vi "Enc_real.vi"(1 "Command":i32, 2 "Encoder":i32, 3 "Encoder_real_in":i32) -> (0 "Encoder_real_out":i32)   [LabVIEW 2015]
panel:
  out "XOR":bool
  out "Cmd > 0?":bool
  out "E(t)-E(t-1)":i32
  out "E(t)-E(t-1) > 0?":bool
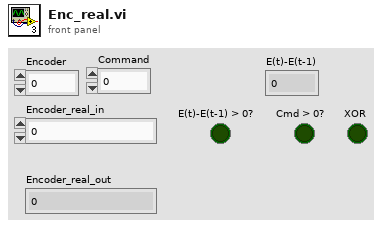
[diagram p1: front panel]
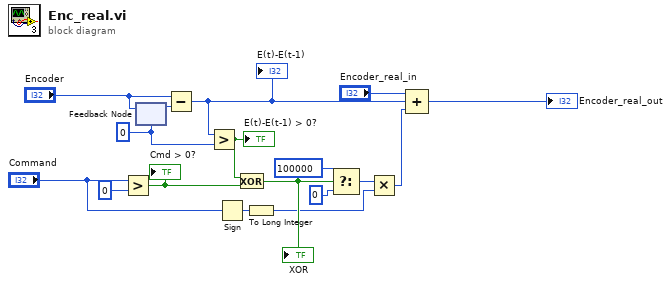
[diagram p0: block diagram]
diagram:
  w17 = 0
  n1 = Greater?(x="Command", y=0) -> (0:w15:bool)
  "Cmd > 0?" <- w15
  n2 = feedback #1(w17) -> (w2:i32)
  n3 = feedback-in #1("Encoder") -> ()
  n4 = Subtract(x="Encoder", y=w2) -> (x-y=w6:i32)
  "E(t)-E(t-1)" <- w6
  n5 = Greater?(x=w6, y=w17) -> (0:w16:bool)
  "E(t)-E(t-1) > 0?" <- w16
  n6 = Sign(1:"Command") -> (0:w12:i32)
  n7 = Exclusive Or(1:w15, 2:w16) -> (0:w14:bool)
  "XOR" <- w14
  n8 = To Long Integer(number=w12) -> (32bit integer=w9:i32)
  n9 = Select(t=100000, s=w14, f=0) -> (s? t:f=w13:i32)
  n10 = Multiply(x=w13, y=w9) -> (x*y=w5:i32)
  n11 = Compound Arithmetic op=ADD("Encoder_real_in", w6, w5) -> (→"Encoder_real_out":i32)
